vi "CRYView Pic Add CurverOutList.vi"(7 "sAction":string, 9 "sName":string, 10 "cCurverOutData":T1) -> ()   [LabVIEW 2013]
uses:
  CRYView Global.vi
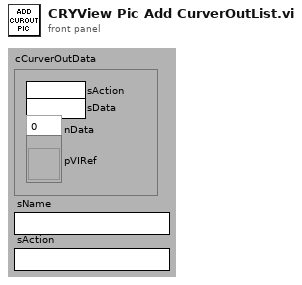
[diagram p1: front panel]
types:
  T1 = cluster{"sAction":string, "sData":string, "nData":i32, "pVIRef":refnum<vi>}
  T2 = cluster{"sAction":string, "sData":string, "nData":i32, "pVIRef":refnum<vi>}[]
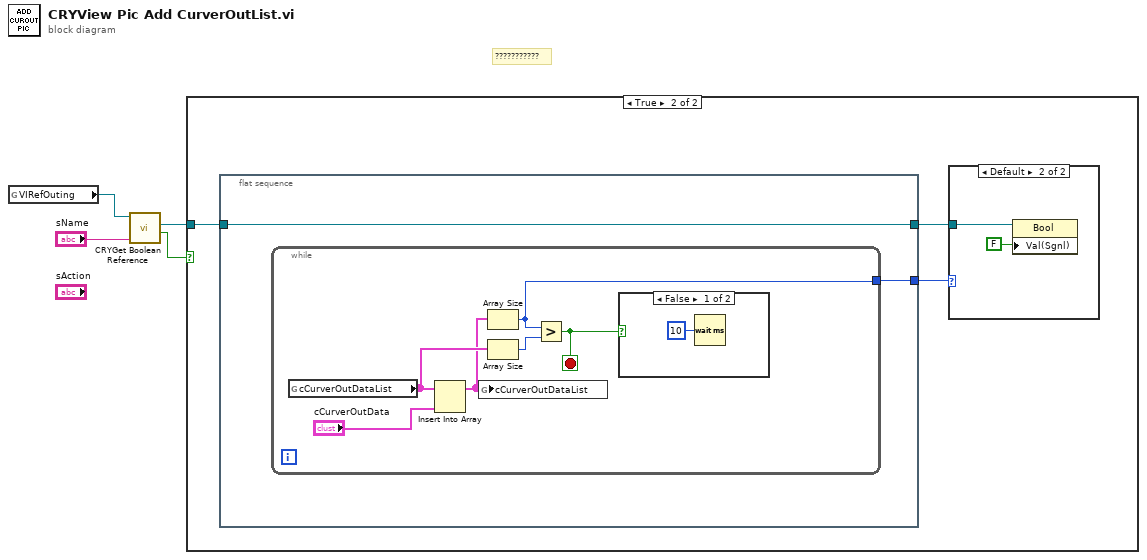
[diagram p0: block diagram]
diagram:
  # "???????????"
  n1 = global read "CRYView Global.vi" "VIRefOuting"() -> (w3:refnum<vi>)
  n2 = call "CRYGet Boolean Reference.vi"("Label Name"="sName", "VI Refnum"=w3) -> ("Exist?"=w1:bool, "Boolean Ref"=w4:refnum<vi>)  [unwired: 7 in, 1 out]
  n3 = case shown="True" w1 {
    tunnel: w4 -> [_ w7]
    frame False {
    }
    frame True {
      n4 = flat-sequence {
        tunnel: w7 -> [w11]
        tunnel: [w11] -> w6
        tunnel: [w10] -> w5
        frame #0 {
          n5 = while {
            tunnel: [w12] -> w10
            stop <- w13 stop-if-true
            n6 = global read "CRYView Global.vi" "cCurverOutDataList"() -> (w16:T2)
            n7 = Insert Into Array(array=w16, new element="cCurverOutData") -> (w15:T2)  [unwired: 1 in]
            n8 = global write "CRYView Global.vi" "cCurverOutDataList"(w15) -> ()
            n9 = Array Size(array=w15) -> (size(s)=w12:i32)
            n10 = Array Size(array=w16) -> (size(s)=w14:i32)
            n11 = Greater?(x=w12, y=w14) -> (0:w13:bool)
            n12 = case shown="False" w13 {
              frame False {
                n13 = Wait (ms)(milliseconds to wait=u32 10) -> ()  [unwired: 1 out]
              }
              frame True {
              }
            }
          }
        }
      }
      n14 = case shown="Default" w5 {
        tunnel: w6 -> [_ w9]
        frame 0 {
        }
        frame Default {
          n15 = property class="Bool"(reference=w9, "Val(Sgnl)"=FALSE) -> ()  [unwired: 1 in, 2 out]
        }
      }
    }
  }
